vi "Get Device Info.vi"(8 "error in (no error)":errorcluster, 11 "Device in":refnum<class "Device.lvclass">) -> (0 "error out":errorcluster, 2 "Device Info":T1, 3 "Device out":refnum<class "Device.lvclass">)   [LabVIEW 2020, in "PicoG-Core.lvlib" / "Device.lvclass"]
uses:
  Device.lvclass
  Device Info.ctl
  Device.lvclass/Device.ctl
  DeployPlatform/DeployPlatform.lvclass
  DeployResource/DeployResource.lvclass
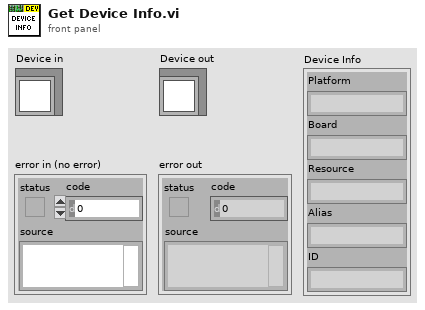
[diagram p1: front panel]
types:
  T1 = typedef "PicoG-Core.lvlib/Device.lvclass/Device Info.ctl" = cluster{"Platform":string, "Board":string, "Resource":string, "Alias":string, "ID":string}
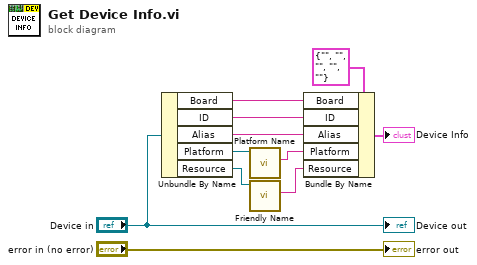
[diagram p0: block diagram]
diagram:
  n1 = Unbundle By Name("Device in") -> ("Board"=w6:string, "ID"=w5:string, "Alias"=w4:string, "Platform"=w9:refnum<class "DeployPlatform.lvclass">, "Resource"=w8:refnum<class "DeployResource.lvclass">)
  n2 = call-dynamic "Platform Name.vi"("DeployTarget in"=w9) -> ("Platform Name"=w3:string)  [unwired: 8 in, 2 out]
  n3 = call-dynamic "Friendly Name.vi"("DeployResource in"=w8) -> ("Friendly Name"=w2:string)  [unwired: 8 in, 2 out]
  n4 = Bundle By Name(cluster=T1 {"Platform"="", "Board"="", "Resource"="", "Alias"="", "ID"=""} ("Device Info"), "Board"=w6, "ID"=w5, "Alias"=w4, "Platform"=w3, "Resource"=w2) -> (→"Device Info":T1)
  "error out" <- "error in (no error)"
  "Device out" <- "Device in"
